vi "Get Handlers.vi"(8 "error in":errorcluster, 11 "Logger in":refnum<class "Logger.lvclass">) -> (0 "error out":errorcluster, 2 "Handlers":refnum<class "Handler.lvclass">[](array[class]), 3 "Logger out":refnum<class "Logger.lvclass">)   [LabVIEW 2020, in "hse-logger.lvlib" / "Logger.lvclass"]
doc: "Returns an array of all Handlers in this logger.\n\n____\nHAMPEL SOFTWARE ENGINEERING v2.0.6 (2021-04-15 11:38)"
uses:
  Logger.lvclass
  Handler/Handler.lvclass
  Logger.lvclass/Logger.ctl
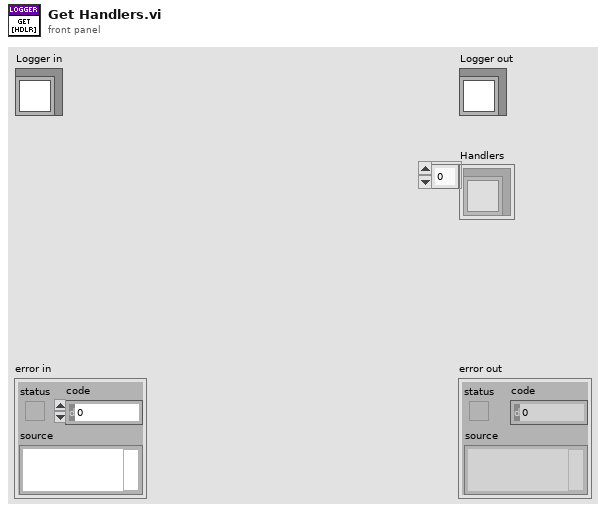
[diagram p1: front panel]
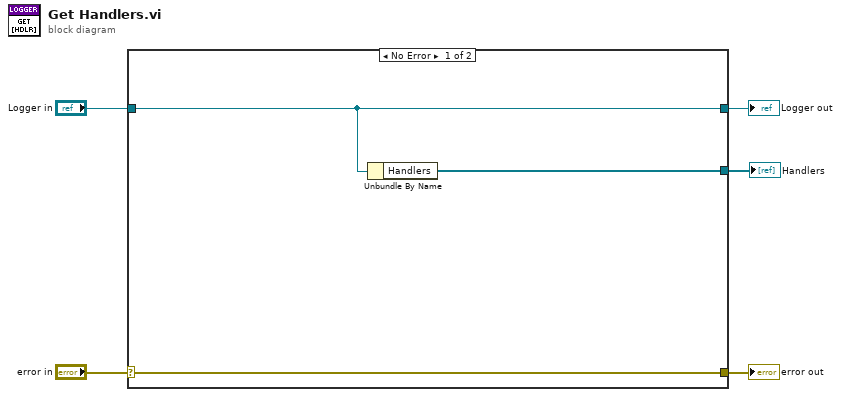
[diagram p0: block diagram]
diagram:
  n1 = case shown="No Error" "error in" {
    selector: "error in" -> [w8 w10]
    tunnel: [w8 w10] -> w4
    tunnel: [w7 w9] -> w2
    tunnel: "Logger in" -> [w7 w9]
    tunnel: [w6 _] -> w1
    frame No Error {
      n2 = Unbundle By Name(w7) -> ("Handlers"=w6:refnum<class "Handler.lvclass">[])
    }
    frame Error {
    }
  }
  "error out" <- w4
  "Logger out" <- w2
  "Handlers" <- w1
